vi "CanRevOne.vi"(7 "CANPort":u16, 8 "data_4":u16, 9 "data_3":u16, 10 "data_2":u16, 11 "data_1":u16) -> (0 "接收数据":u16[](array[numeric]), 2 "成功？":bool)   [LabVIEW 2010]
uses:
  全局量/全局_配置.vi
panel:
  out "开始时间":dbl format="%#.0f"
  in  "字符串":string
  out "Error out":errorcluster {"code" format="%.0x"}
  in  "ReadTimeOut":u32=3000 caption="ms"
  in  "Synchronization":i32(ring)=1 items=["Synchronization"=1, "Asynchronization"=0]
  # "从0开始"
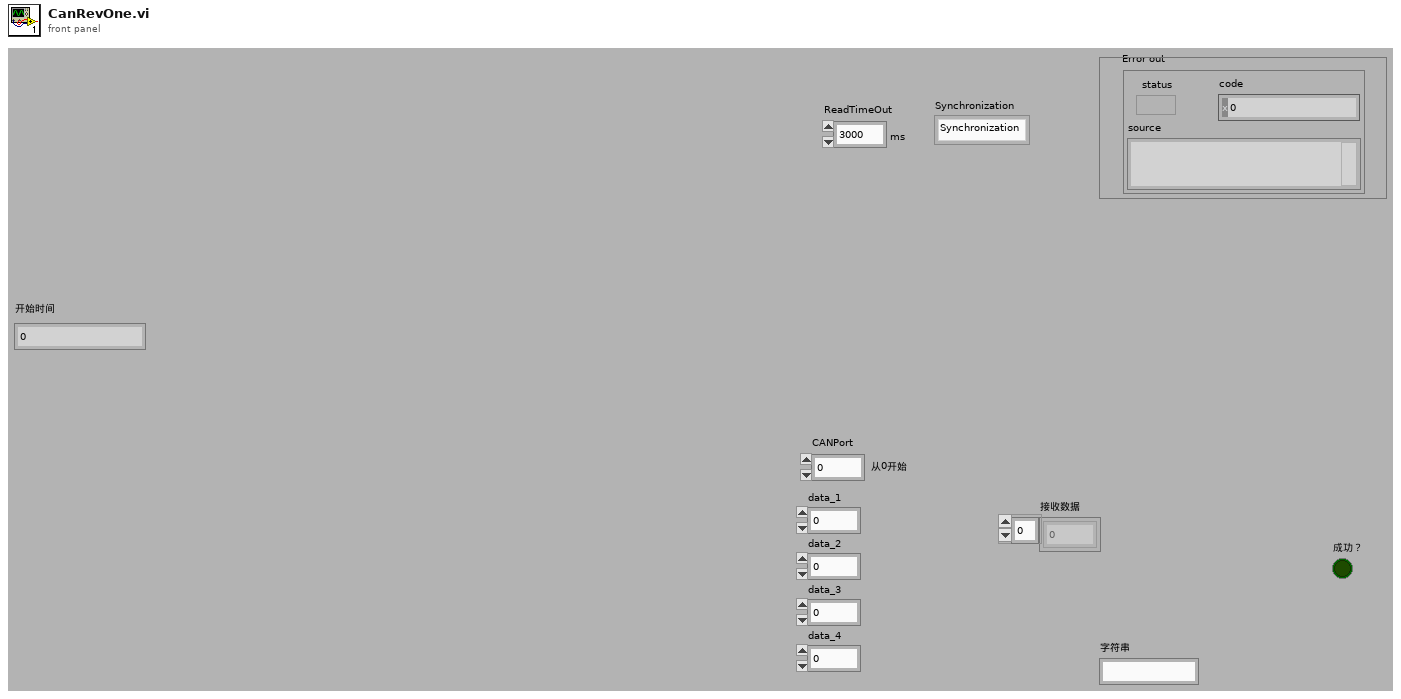
[diagram p1: front panel]
types:
  T1 = cluster{"Internal":u32, "InternalHigh":u32, "Offset":u32, "OffsetHigh":u32, "hEvent":u32}
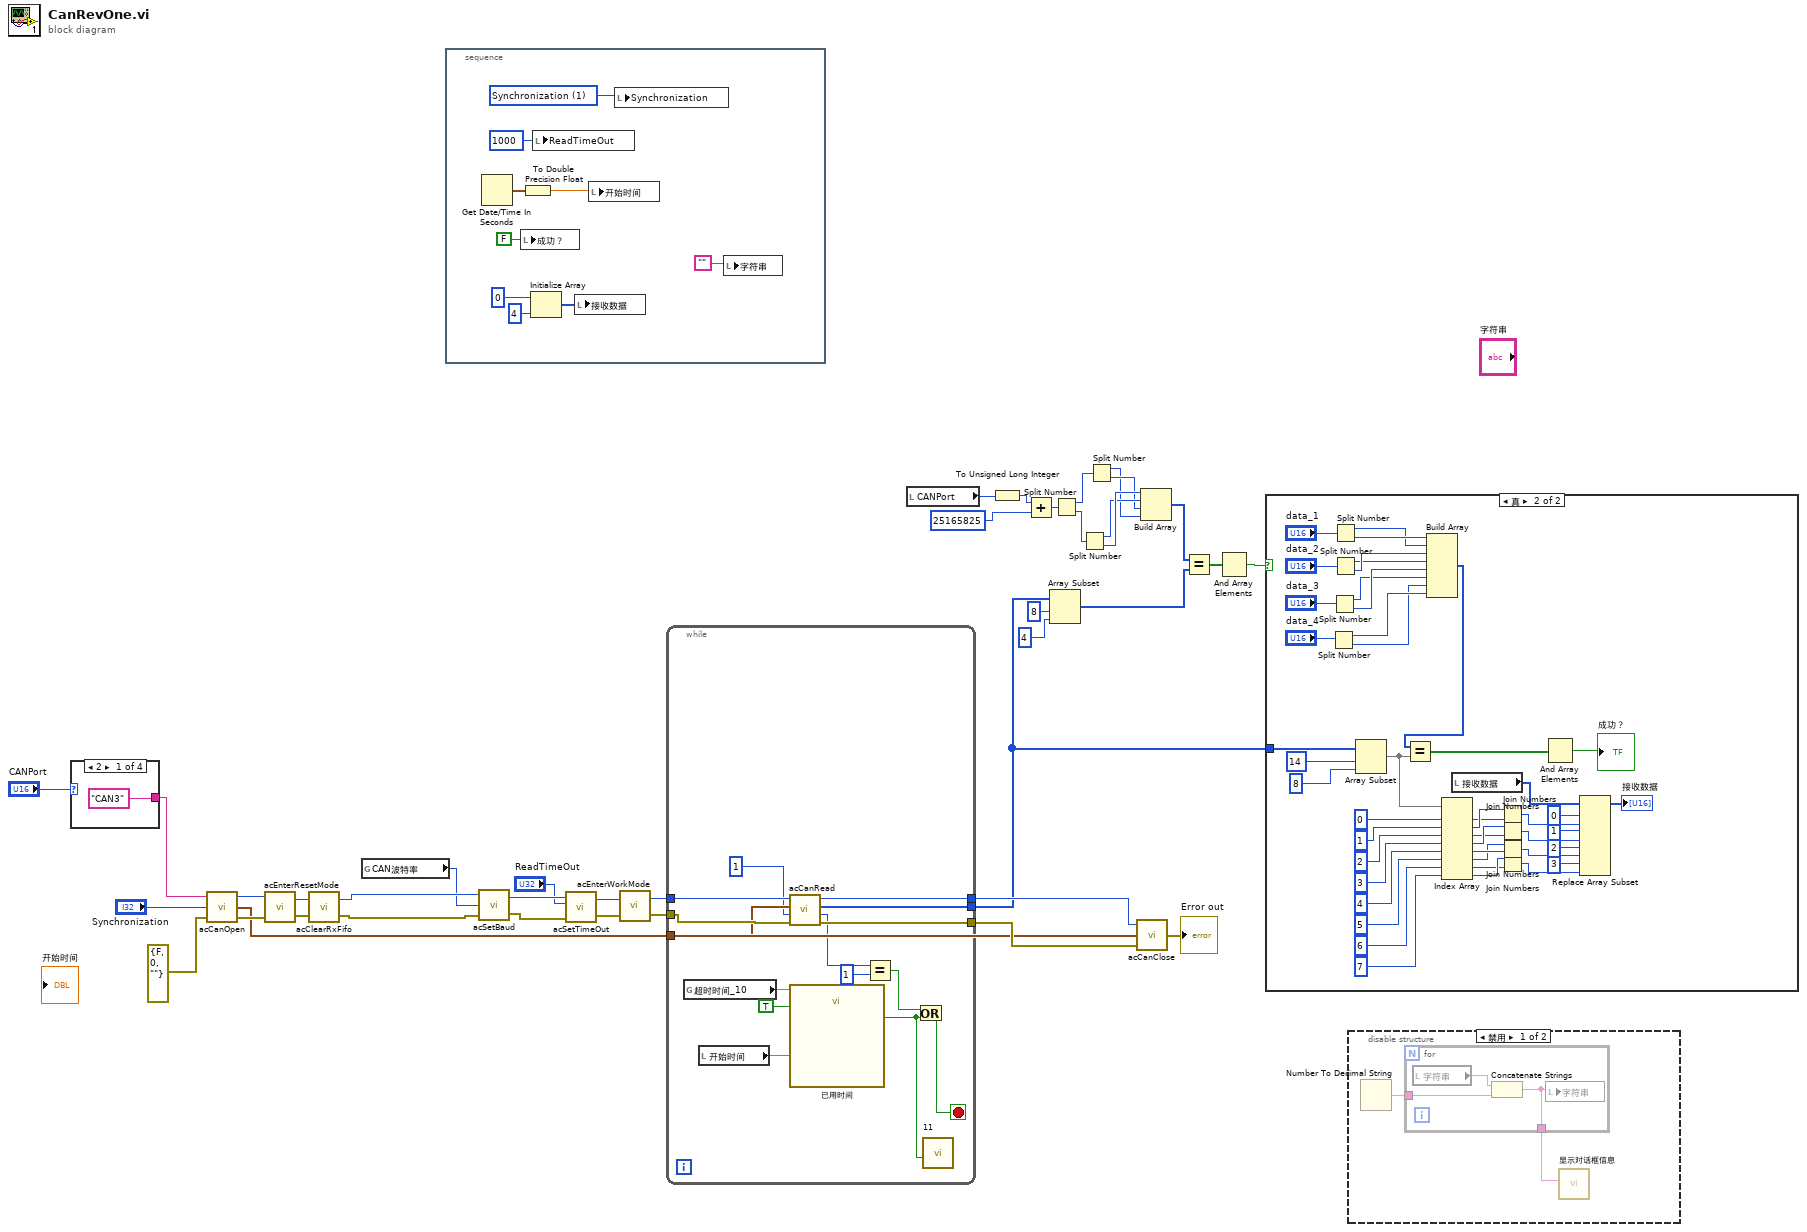
[diagram p0: block diagram]
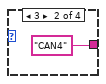
[diagram p4: hidden frame]
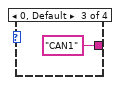
[diagram p5: hidden frame]
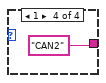
[diagram p6: hidden frame]
diagram:
  n1 = case shown="2" "CANPort" {
    tunnel: ["CAN3" "CAN4" "CAN1" "CAN2"] -> w20
    frame 2 {
    }
    frame 3 {
    }
    frame 0, Default {
    }
    frame 1 {
    }
  }
  n2 = call "acCanOpen.vi"("Error in"=errorcluster {"status"=FALSE, "code"=0, "source"=""}, "Synchronization"="Synchronization", "CANPort"=w20) -> ("Error out"=w35:errorcluster, "Overlapped"=w3:T1, "Handle"=w36:u32)
  n3 = call "acEnterResetMode.vi"("Error in"=w35, "Handle  in"=w36) -> ("Error out"=w29:errorcluster, "Handle out"=w28:u32)
  n4 = call "acClearRxFifo.vi"("Error in"=w29, "Handle  in"=w28) -> ("Error out"=w26:errorcluster, "Handle out"=w27:u32)
  n5 = global read "全局_配置.vi" "CAN波特率"() -> (w1:u16)
  n6 = stacked-sequence {
    frame #0 {
      w50 = 1 items=["Synchronization"=1, "Asynchronization"=0] ("Synchronization")
      n7 = Get Date/Time In Seconds() -> (seconds since 1Jan1904=w45:timestamp)
      n8 = local write "成功？"(FALSE ("成功？")) -> ()
      n9 = To Double Precision Float(number=w45) -> (double precision float=w44:dbl)
      n10 = Initialize Array(u16 0, 4 ("维数大小")) -> (w47:u16[])
      n11 = local write "ReadTimeOut"(u32 1000 ("ReadTimeOut")) -> ()
      n12 = local write "接收数据"(w47) -> ()
      n13 = local write "开始时间"(w44) -> ()
      n14 = local write "Synchronization"(w50) -> ()
      n15 = local write "字符串"("") -> ()
    }
  }
  n16 = call "acSetBaud.vi"("Error in"=w26, "Baudrate"=w1, "Handle  in"=w27) -> ("Error out"=w31:errorcluster, "Handle out"=w32:u32)
  n17 = call "acSetTimeOut.vi"("Error in"=w31, "Read TimeOut"="ReadTimeOut", "Handle  in"=w32) -> ("Error out"=w24:errorcluster, "Handle out"=w25:u32)  [unwired: 1 in]
  n18 = call "acEnterWorkMode.vi"("Error in"=w24, "Handle  in"=w25) -> ("Error out"=w22:errorcluster, "Handle out"=w23:u32)
  n19 = while {
    tunnel: [w67] -> w38
    tunnel: [w66] -> w37
    tunnel: w23 -> [w65]
    tunnel: w22 -> [w64]
    tunnel: w3 -> [w63]
    tunnel: [w61] -> w2
    stop <- w54 stop-if-true
    n20 = global read "全局_配置.vi" "超时时间_10"() -> (w59:dbl)
    n21 = local read "开始时间"() -> (w60:dbl)
    n22 = call "acCanRead.vi"("Error in"=w64, "ReadCount"=u32 1 ("接收CAN帧数 2"), "Overlapped"=w63, "Handle  in"=w65) -> ("Error out"=w66:errorcluster, "NumberOfRead"=w57:u32, "MSG"=w61:u8[], "Handle out"=w67:u32)
    n23 = call "已用时间"("Time Target (s)"=w59, "Reset"=TRUE, "Set Start Time (s)"=w60) -> ("Time has Elapsed"=w53:bool)  [unwired: 9 in, 7 out]
    n24 = Equal?(x=w57, y=u32 1) -> (x = y?=w55:bool)
    n25 = Or(x=w55, y=w53) -> (x .or. y?=w54:bool)
    n26 = call "11"("Enable"=w53) -> ()  [unwired: 9 in, 2 out]
  }
  n27 = local read "CANPort"() -> (w4:u16)
  n28 = To Unsigned Long Integer(number=w4) -> (unsigned 32bit integer=w18:u32)
  n29 = Add(x=w18, y=u32 25165825) -> (x+y=w17:u32)
  n30 = Array Subset(array=w2, index=8 ("索引"), length=4 ("长度")) -> (w7:u8[])
  n31 = Split Number(x=w17) -> (hi(x)=w16:u16, lo(x)=w15:u16)
  n32 = Split Number(x=w15) -> (hi(x)=w13:u8, lo(x)=w14:u8)
  n33 = Split Number(x=w16) -> (hi(x)=w11:u8, lo(x)=w12:u8)
  n34 = call "acCanClose.vi"("Error in"=w37, "Overlapped"=w3, "Handle  in"=w38) -> ("Error out"=→"Error out":errorcluster)
  n35 = Build Array(w14, w13, w12, w11) -> (w8:u8[])
  n36 = Equal?(x=w8, y=w7) -> (x = y?=w6:bool[])
  n37 = And Array Elements(Boolean array=w6) -> (logical AND=w5:bool)
  n38 = case shown="真" w5 {
    tunnel: w2 -> [_ w68]
    frame False {
    }
    frame True {
      n39 = Split Number(x="data_4") -> (hi(x)=w101:u8, lo(x)=w100:u8)
      n40 = Split Number(x="data_3") -> (hi(x)=w102:u8, lo(x)=w103:u8)
      n41 = Split Number(x="data_1") -> (hi(x)=w106:u8, lo(x)=w107:u8)
      n42 = Split Number(x="data_2") -> (hi(x)=w104:u8, lo(x)=w105:u8)
      n43 = Array Subset(array=w68, index=14 ("索引"), length=8 ("长度")) -> (w70:u8[])
      n44 = Build Array(w107, w106, w105, w104, w103, w102, w100, w101) -> (w69:u8[])
      n45 = Equal?(x=w69, y=w70) -> (x = y?=w112:bool[])
      n46 = Index Array(array=w70, index #1=0 ("索引"), index #2=1 ("索引"), index #3=2 ("索引"), index #4=3 ("索引"), index #5=4 ("索引"), index #6=5 ("索引"), index #7=6 ("索引"), index #8=7 ("索引")) -> (element #1=w87:u8, element #2=w88:u8, element #3=w85:u8, element #4=w86:u8, element #5=w84:u8, element #6=w83:u8, element #7=w81:u8, element #8=w82:u8)
      n47 = local read "接收数据"() -> (w80:u16[])
      n48 = Join Numbers(hi=w88, lo=w87) -> ((hi.lo)=w77:u16)
      n49 = Join Numbers(hi=w86, lo=w85) -> ((hi.lo)=w75:u16)
      n50 = Join Numbers(hi=w83, lo=w84) -> ((hi.lo)=w73:u16)
      n51 = Join Numbers(hi=w82, lo=w81) -> ((hi.lo)=w71:u16)
      n52 = And Array Elements(Boolean array=w112) -> (logical AND=→"成功？":bool)
      n53 = Replace Array Subset(array=w80, new element #1=w77, index #1=0 ("索引"), new element #2=w75, index #2=1 ("索引"), new element #3=w73, index #3=2 ("索引"), new element #4=w71, index #4=3 ("索引")) -> (→"接收数据":u16[])
    }
  }
  n54 = disable-structure shown="禁用" {
    frame Disabled {
      n55 = Number To Decimal String() -> (decimal integer string=w114:string)  [unwired: 2 in]
      n56 = for {
        tunnel: w114 -> [w116]
        tunnel: [w115] -> w113
        n57 = local read "字符串"() -> (w117:string)
        n58 = Concatenate Strings(w117, w116) -> (w115:string)
        n59 = local write "字符串"(w115) -> ()
      }
      n60 = call "显示对话框信息"("Message"=w113) -> ()  [unwired: 9 in, 2 out]
    }
    frame Enabled {
    }
  }
